vi "Configure Hardware.vi"(8 "error in (no error)":errorcluster, 11 "Hardware Resources in":T1) -> (0 "error out":errorcluster, 3 "Hardware Resources out":T1)   [LabVIEW 2019, in "Acquisition.lvlib"]
doc: "Configure the hardware."
uses:
  Acquisition.lvlib
  Hardware Configuration.ctl
  <vilib>/DAQmx/create/channels.llb/DAQmx Create Channel (AI-Voltage-Basic).vi
  <vilib>/DAQmx/configure/timing.llb/DAQmx Timing (Sample Clock).vi
  <vilib>/DAQmx/configure/trigger.llb/DAQmx Start Trigger (Analog Edge).vi
  <vilib>/DAQmx/create/channels.llb/DAQmx Create Channel (AO-Current-Basic).vi
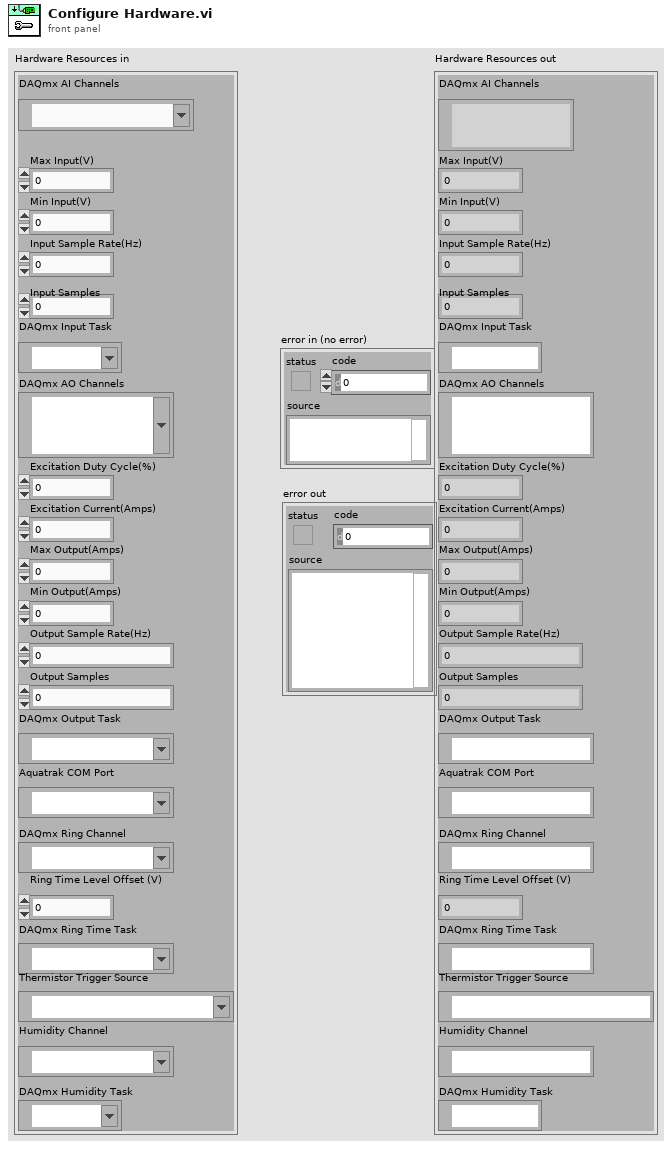
[diagram p1: front panel]
types:
  T1 = typedef "Acquisition.lvlib/Hardware Configuration.ctl" = cluster{"DAQmx AI Channels":tag, "Max Input(V)":dbl, "Min Input(V)":dbl, "Input Sample Rate(Hz)":dbl, "Input Samples":dbl, "DAQmx Input Task":refnum<k21>, "DAQmx AO Channels":tag, "Excitation Duty Cycle(%)":dbl, "Excitation Current(Amps)":dbl, "Max Output(Amps)":dbl, "Min Output(Amps)":dbl, "Output Sample Rate(Hz)":dbl, "Output Samples":dbl, "DAQmx Output Task":refnum<k21>, "Aquatrak COM Port":refnum<visa-resource-name>, "DAQmx Ring Channel":tag, "Ring Time Level Offset (V)":dbl, "DAQmx Ring Time Task":refnum<k21>, "Thermistor Trigger Source":tag, "Humidity Channel":tag, "DAQmx Humidity Task":refnum<k21>}
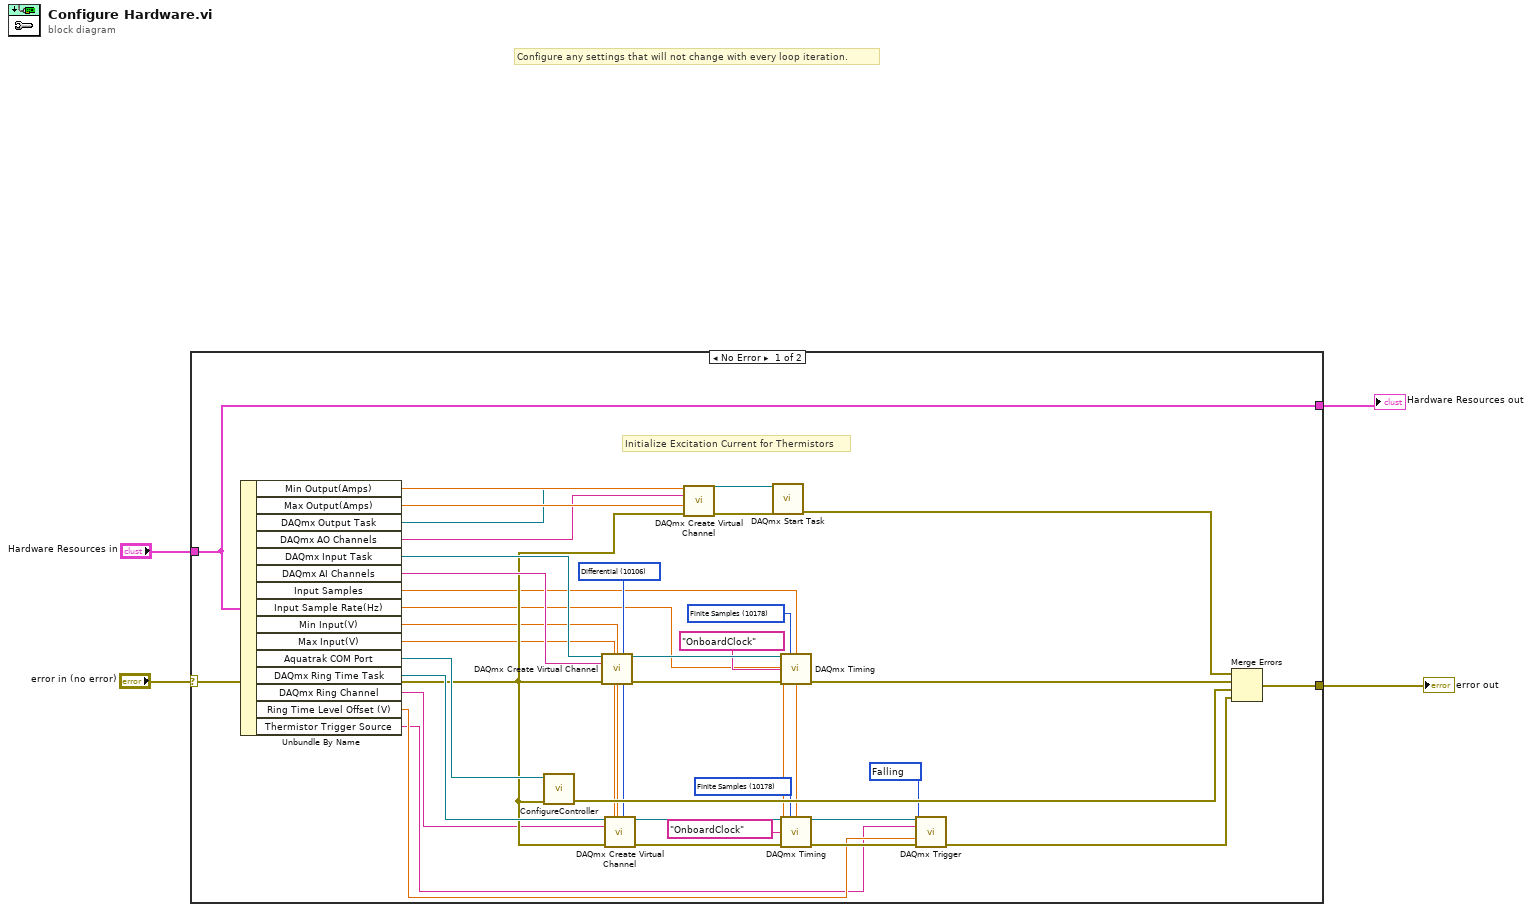
[diagram p0: block diagram]
diagram:
  # "Configure any settings that will not change with every loop iteration."
  n1 = case shown="No Error" "error in (no error)" {
    selector: "error in (no error)" -> [w22 w41]
    tunnel: [w34 w41] -> w3
    tunnel: "Hardware Resources in" -> [w27 w42]
    tunnel: [w27 w42] -> w1
    frame No Error {
      w7 = 10171 items=["Rising"=10280, "Falling"=10171] ("slope")
      w16 = 10178 items=["Finite Samples"=10178, "Continuous Samples"=10123, "Hardware Timed Single Point"=12522] ("sample mode")
      w17 = 10106 items=["default"=-1, "RSE"=10083, "NRSE"=10078, "Differential"=10106, "Pseudodifferential"=12529] ("input terminal configuration")
      w26 = 10178 items=["Finite Samples"=10178, "Continuous Samples"=10123, "Hardware Timed Single Point"=12522] ("sample mode")
      # "Initialize Excitation Current for Thermistors"
      n2 = Unbundle By Name(w27) -> ("Min Output(Amps)"=w39:dbl, "Max Output(Amps)"=w38:dbl, "DAQmx Output Task"=w37:refnum<k21>, "DAQmx AO Channels"=w36:tag, "DAQmx Input Task"=w40:refnum<k21>, "DAQmx AI Channels"=w35:tag, "Input Samples"=w15:dbl, "Input Sample Rate(Hz)"=w14:dbl, "Min Input(V)"=w20:dbl, "Max Input(V)"=w21:dbl, "Aquatrak COM Port"=w29:refnum<visa-resource-name>, "DAQmx Ring Time Task"=w23:refnum<k21>, "DAQmx Ring Channel"=w5:tag, "Ring Time Level Offset (V)"=w8:dbl, "Thermistor Trigger Source"=w6:tag)
      n3 = call "ConfigureController.vi"("error in (no error)"=w22, "VISA resource name"=w29) -> ("error out"=w28:errorcluster)  [unwired: 8 in, 1 out]
      n4 = call-poly <vilib>:"DAQmx Create Virtual Channel.vi"("task in"=w40, "maximum value"=w21, "minimum value"=w20, "input terminal configuration"=w17, "physical channels"=w35, "error in"=w22) -> ("task out"=w33:refnum<k21>, "error out"=w24:errorcluster)  [unwired: 8 in]
      n5 = call-poly <vilib>:"DAQmx Create Virtual Channel.vi"("task in"=w23, "maximum value"=w21, "minimum value"=w20, "input terminal configuration"=w17, "physical channels"=w5, "error in"=w22) -> ("task out"=w18:refnum<k21>, "error out"=w13:errorcluster)  [unwired: 8 in]
      n6 = call-poly <vilib>:"DAQmx Create Virtual Channel.vi"("task in"=w37, "maximum value"=w38, "minimum value"=w39, "physical channels"=w36, "error in"=w22) -> ("task out"=w32:refnum<k21>, "error out"=w31:errorcluster)  [unwired: 9 in]
      n7 = call <vilib>:"DAQmx Start Task.vi"("task/channels in"=w32, "error in"=w31) -> ("error out"=w30:errorcluster)  [unwired: 12 in, 1 out]
      n8 = call-poly <vilib>:"DAQmx Timing.vi"("task/channels in"=w33, "sample mode"=w26, "samples per channel"=w15, "rate"=w14, "source"=tag "OnboardClock", "error in"=w24) -> ("error out"=w10:errorcluster)  [unwired: 8 in, 1 out]
      n9 = call-poly <vilib>:"DAQmx Timing.vi"("task/channels in"=w18, "sample mode"=w16, "samples per channel"=w15, "rate"=w14, "source"=tag "OnboardClock", "error in"=w13) -> ("task out"=w12:refnum<k21>, "error out"=w11:errorcluster)  [unwired: 8 in]
      n10 = call-poly <vilib>:"DAQmx Trigger.vi"("task/channels in"=w12, "source"=w6, "slope"=w7, "level"=w8, "error in"=w11) -> ("error out"=w9:errorcluster)  [unwired: 9 in, 1 out]
      n11 = Merge Errors(w30, w10, w28, w9) -> (w34:errorcluster)
    }
    frame Error {
    }
  }
  "Hardware Resources out" <- w1
  "error out" <- w3
